vi "update_issue_display_date.vi"(8 "in collection":bool, 9 "issues in":i32, 10 "Cover Date":timestamp, 11 "issues in":T1[](array[typedef]) {"display_date" format="%<%x>T"}) -> (2 "issue":T1 {"display_date" format="%<%x>T"}, 3 "issues out":T1[](array[typedef]) {"display_date" format="%<%x>T"})   [LabVIEW 2024]
uses:
  CV_RESTful_Library/typedefs/local_issue--cluster.ctl
  CV_RESTful_Library/typedefs/cv_issue.generic_credit--cluster.ctl
  CV_RESTful_Library/typedefs/cv_issue.associated_image--cluster.ctl
  CV_RESTful_Library/typedefs/cv_issue.person_credit--cluster.ctl
  CV_RESTful_Library/CV_RESTful_Lib.lvlib
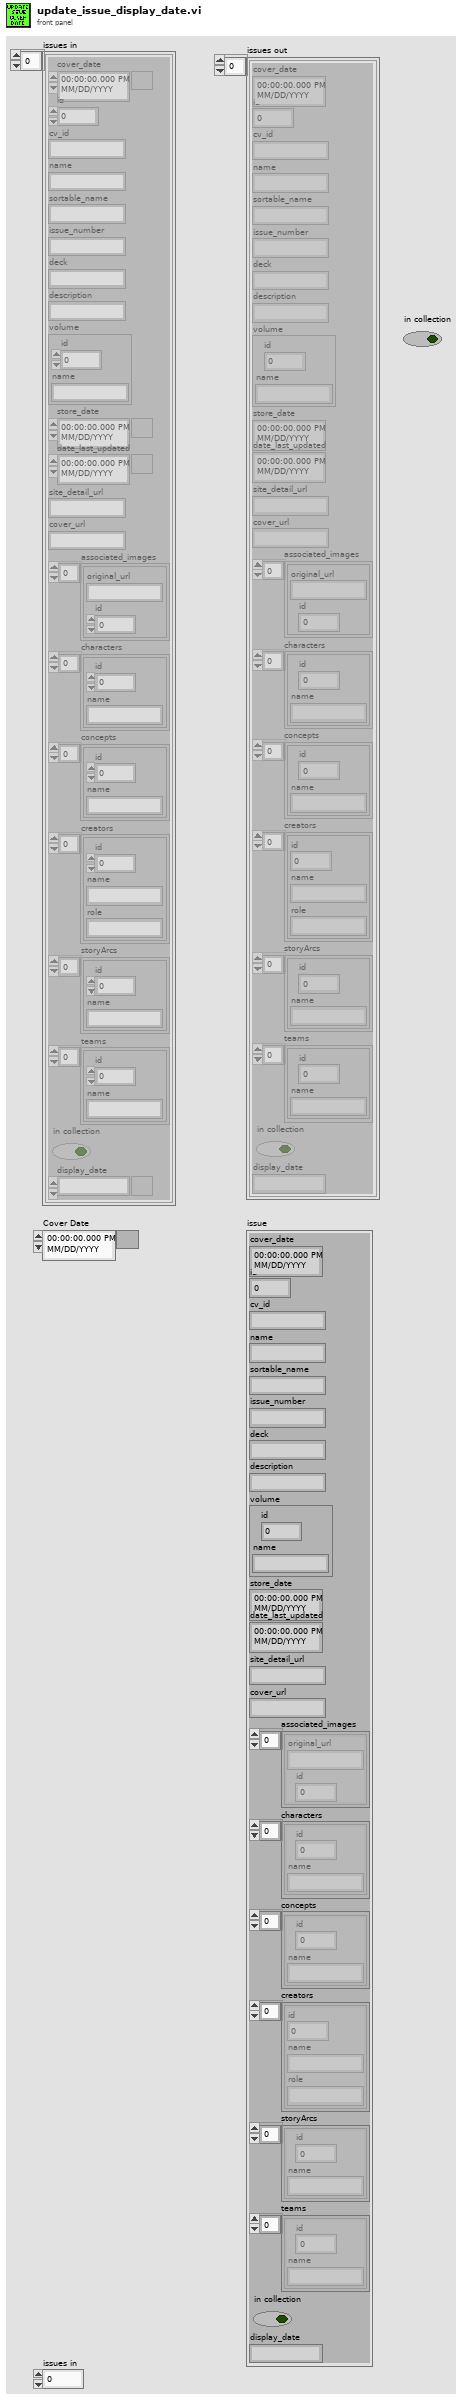
[diagram p1: front panel]
types:
  T1 = typedef "CV_RESTful_Lib.lvlib/local_issue--cluster.ctl" = cluster{"cover_date":timestamp, "id":i32, "cv_id":string, "name":string, "sortable_name":string, "issue_number":string, "deck":string, "description":string, "volume":T2, "store_date":timestamp, "date_last_updated":timestamp, "site_detail_url":string, "cover_url":string, "associated_images":T3[], "characters":T2[], "concepts":T2[], "creators":T4[], "storyArcs":T2[], "teams":T2[], "in collection":bool, "display_date":timestamp}
  T2 = typedef "CV_RESTful_Lib.lvlib/cv_issue.generic_credit--cluster.ctl" = cluster{"id":i32, "name":string}
  T3 = typedef "CV_RESTful_Lib.lvlib/cv_issue.associated_image--cluster.ctl" = cluster{"original_url":string, "id":i32}
  T4 = typedef "CV_RESTful_Lib.lvlib/cv_issue.person_credit--cluster.ctl" = cluster{"id":i32, "name":string, "role":string}
  T5 = typedef "LVDateTimeRec.ctl" = cluster{"fractional second":dbl, "second":i32, "minute":i32, "hour":i32, "day of month":i32, "month":i32, "year":i32, "day of week":i32, "day of year":i32, "DST":i32}
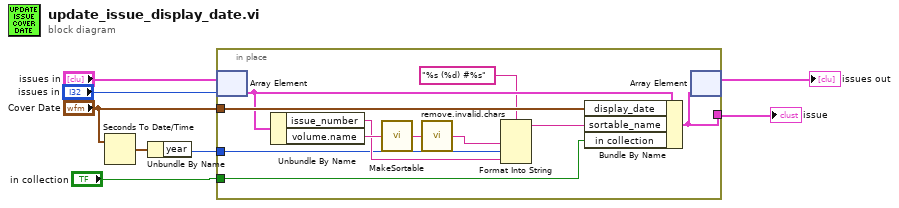
[diagram p0: block diagram]
diagram:
  n1 = Seconds To Date/Time(time stamp (now)="Cover Date") -> (date time rec=w6:T5)  [unwired: 1 in]
  n2 = Unbundle By Name(w6) -> ("year"=w8:i32)
  n3 = in-place {
    in-place-border: "Cover Date" -> [w19]
    in-place-border: [w18] -> w5
    in-place-border: w8 -> [w11]
    in-place-border: "in collection" -> [w9]
    n4 = in-place-array #1("issues in", "issues in") -> (w17:T1)
    n5 = Unbundle By Name(w17) -> ("issue_number"=w12:string, "volume.name"=w13:string)
    n6 = call "MakeSortable.vi"("string in"=w13) -> ("string out"=w15:string)
    n7 = call "remove.invalid.chars.vi"("string in"=w15) -> ("string out"=w14:string)
    n8 = Format Into String(format string="%s (%d) #%s", w14, w11, w12) -> (resulting string=w16:string)  [unwired: 2 in, 1 out]
    n9 = Bundle By Name(cluster=w17, "display_date"=w19, "sortable_name"=w16, "in collection"=w9) -> (w18:T1)
    n10 = in-place-array #1(w18) -> (→"issues out":T1[])  [unwired: 1 out]
  }
  "issue" <- w5
